vi "Read Plugin INI.vi"(8 "error in (no error)":errorcluster, 11 "INI file":path) -> (0 "error out":errorcluster, 3 "Plugin Details":T1={"Plugin Name"="", "Controller Type"=enum."Invalid", "Control Panel Path"=path "", "Plugin Type"=enum."Optimizer"})   [LabVIEW 2020, in "Plugin Manager.lvlib"]
uses:
  Plugin Manager.lvlib
  Plugin Details.ctl
  Plugin Servers/Controller/Controller Type.ctl
  Plugin Types.ctl
  <vilib>/Utility/config.llb/NI_LVConfig.lvlib
  Plugin Servers/Controller/Generic Plugin.lvclass
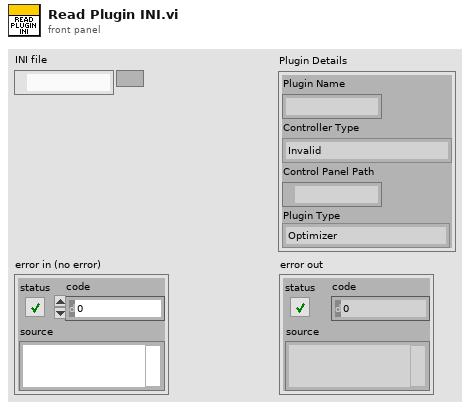
[diagram p1: front panel]
types:
  T1 = typedef "Plugin Manager.lvlib/Plugin Details.ctl" = cluster{"Plugin Name":string, "Controller Type":T2, "Control Panel Path":path, "Plugin Type":T3}
  T2 = typedef "Generic Plugin.lvclass/Controller Type.ctl" = enum16{"Invalid", "Temperature Controller", "Pump Controller", "Generic Optimizer", "LC Parser"}
  T3 = typedef "Plugin Manager.lvlib/Plugin Types.ctl" = enum16{"Invalid", "Optimizer", "Analyzer", "Hardware"}
  T4 = typedef "NI_LVConfig.lvlib/Config Data RefNum.ctl" = refnum<k1>
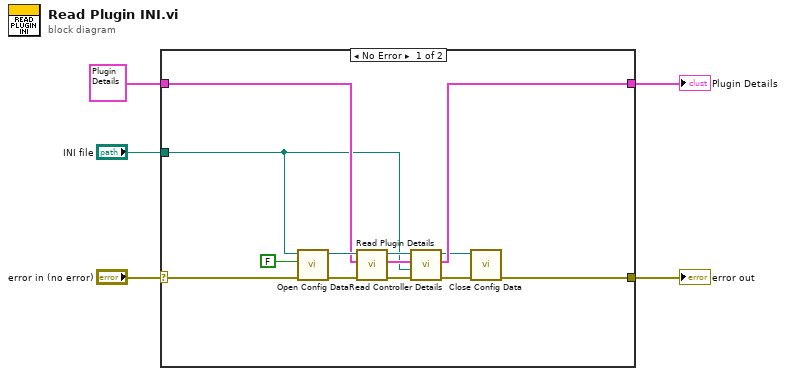
[diagram p0: block diagram]
diagram:
  n1 = case shown="No Error" "error in (no error)" {
    selector: "error in (no error)" -> [w18 w20]
    tunnel: [w8 w20] -> w4
    tunnel: "INI file" -> [w6 _]
    tunnel: T1 {"Plugin Name"="", "Controller Type"=enum."Invalid", "Control Panel Path"=path "", "Plugin Type"=enum."Optimizer"} ("Plugin Details") -> [w11 w19]
    tunnel: [w9 w19] -> w1
    frame No Error {
      n2 = call <vilib>:"Open Config Data.vi"("error in (no error)"=w18, "create file if necessary (T)"=FALSE, "configuration file path"=w6) -> ("error out"=w15:errorcluster, "refnum"=w13:T4)  [unwired: 6 in, 1 out]
      n3 = call "Read Plugin Details.vi"("error in (no error)"=w15, "Plugin Details in"=w11, "Plugin File Refnum in"=w13) -> ("error out"=w14:errorcluster, "Plugin Details out"=w10:T1, "Plugin File Refnum out"=w12:T4)  [unwired: 6 in]
      n4 = call "Read Controller Details.vi"("error in (no error)"=w14, "Plugin File Path"=w6, "Plugin Details in"=w10, "Refnum in"=w12) -> ("error out"=w17:errorcluster, "Plugin Details out 2"=w9:T1, "refnum out"=w7:T4)  [unwired: 5 in]
      n5 = call <vilib>:"Close Config Data.vi"("error in (no error)"=w17, "refnum"=w7) -> ("error out"=w8:errorcluster)  [unwired: 8 in, 1 out]
    }
    frame Error {
    }
  }
  "error out" <- w4
  "Plugin Details" <- w1
